vi "MongoDB.EnumerateResult.vi"(8 "error in (no error)":errorcluster, 11 "MongoDB.Cursor":refnum<k24>) -> (0 "error out":errorcluster, 3 "Array":string[](array[string]))   [LabVIEW 2014]
uses:
  C:/Users/Richard/Documents/GitHub/mongo-labview-driver/CSharp/bin/MongoDB.Driver.Legacy.dll
  CSharp/bin/MongoDB.Driver.Legacy.dll
  C:/Users/Richard/Documents/GitHub/mongo-labview-driver/CSharp/bin/MongoDB.Bson.dll
  CSharp/bin/MongoDB.Bson.dll
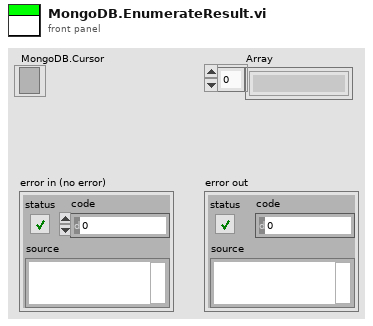
[diagram p1: front panel]
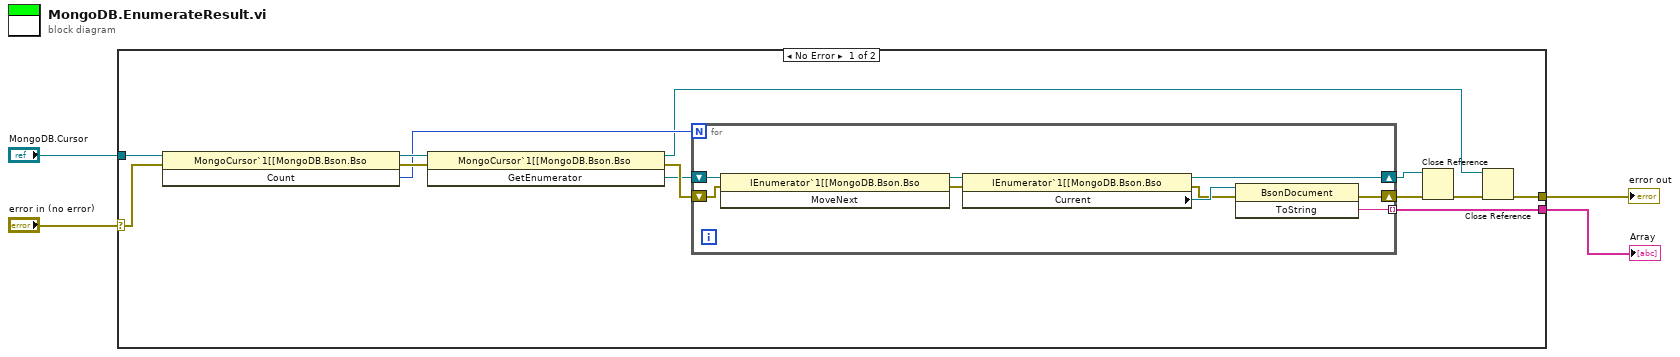
[diagram p0: block diagram]
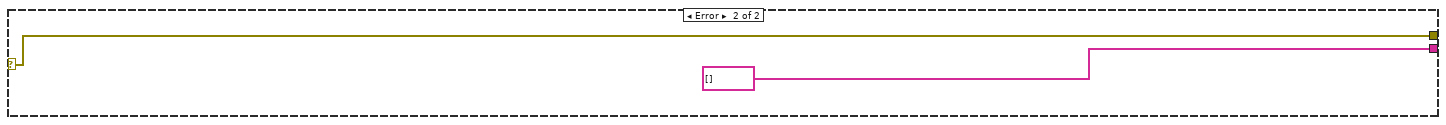
[diagram p2: hidden frame]
diagram:
  n1 = case shown="No Error" "error in (no error)" {
    selector: "error in (no error)" -> [w10 w28]
    tunnel: [w6 w28] -> w4
    tunnel: [w15 string[] []] -> w3
    tunnel: "MongoDB.Cursor" -> [w11 _]
    frame No Error {
      n2 = invoke class="MongoCursor`1[[MongoDB.Bson.Bso" method="Count"(reference=w11, error in=w10) -> (reference out=w17:refnum<k24>, error out=w16:errorcluster, "Count"=w12:i64)  [unwired: 1 in]
      n3 = invoke class="MongoCursor`1[[MongoDB.Bson.Bso" method="GetEnumerator"(reference=w17, error in=w16) -> (reference out=w9:refnum<k24>, error out=w14:errorcluster, "GetEnumerator"=w13:refnum<k24>)  [unwired: 1 in]
      n4 = for {
        N: w12 -> [_]
        shift-right: [w20] -> w5
        shift-left: w13 -> [w23]
        tunnel: [w21] -> w15 mode=indexing
        shift-right: [w18] -> w8
        shift-left: w14 -> [w25]
        n5 = invoke class="IEnumerator`1[[MongoDB.Bson.Bso" method="MoveNext"(reference=w23, error in=w25) -> (reference out=w26:refnum<k24>, error out=w24:errorcluster)  [unwired: 1 in, 1 out]
        n6 = property class="IEnumerator`1[[MongoDB.Bson.Bso"(reference=w26, error in=w24) -> (reference out=w20:refnum<k24>, error out=w19:errorcluster, "Current"=w22:refnum<k24>)
        n7 = invoke class="BsonDocument" method="ToString"(reference=w22, error in=w19) -> (error out=w18:errorcluster, "ToString"=w21:string)  [unwired: 1 in, 1 out]
      }
      n8 = Close Reference(reference=w5, error in (no error)=w8) -> (error out=w7:errorcluster)
      n9 = Close Reference(reference=w9, error in (no error)=w7) -> (error out=w6:errorcluster)
    }
    frame Error {
    }
  }
  "error out" <- w4
  "Array" <- w3
